vi "介面改良.vi"() -> ()   [LabVIEW 2022 SP3]
uses:
  <vilib>/httpClient/LabVIEWHTTPClient.lvlib
panel:
  in  "stop":bool
  in  "開始運作":bool
  out "異常指示燈":bool
  out "目前溫度":dbl
  in  "-10":bool
  in  "-5":bool
  in  "+5":bool
  in  "+10":bool
  out "目標溫度控制":string
  in  "溫差容許值":dbl
  in  "目標溫度":dbl
  in  "進階選單":bool
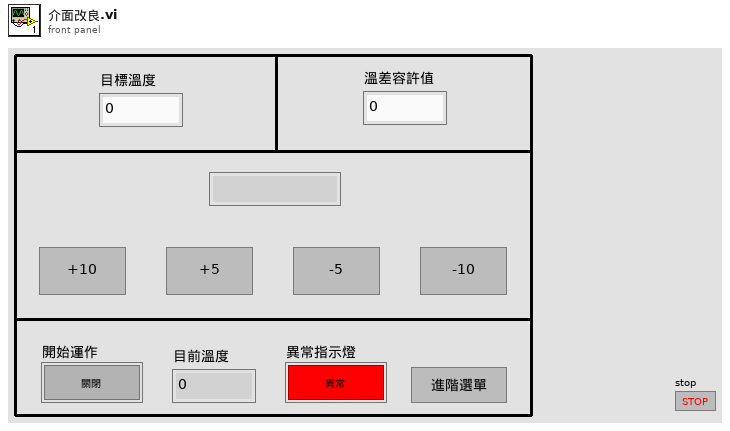
[diagram p1: front panel]
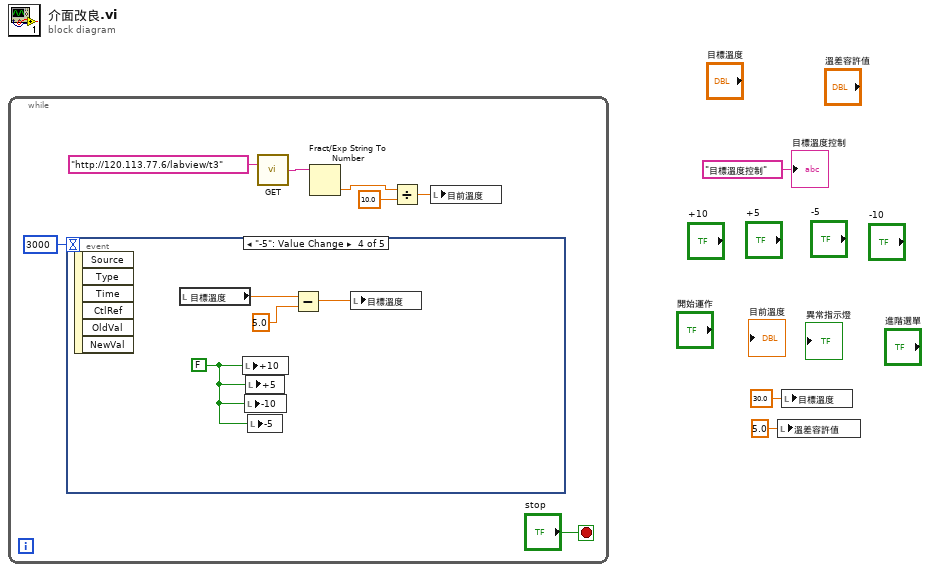
[diagram p0: block diagram]
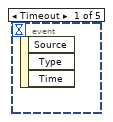
[diagram p2: hidden frame]
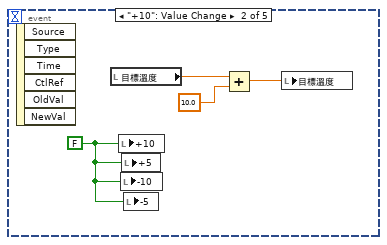
[diagram p3: hidden frame]
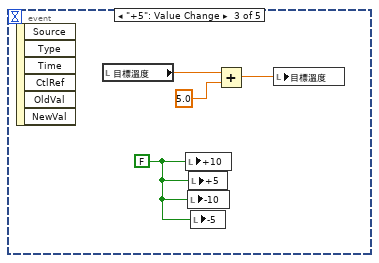
[diagram p4: hidden frame]
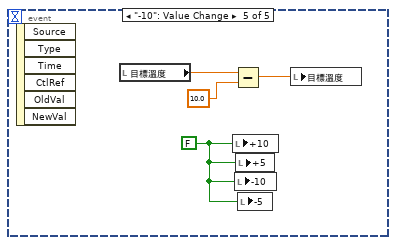
[diagram p5: hidden frame]
diagram:
  n1 = while {
    stop <- "stop" stop-if-true
    n2 = event shown="[3] \"-5\": Value Change" {
      selector: _ -> [_ _ _ _ _]
      dyn-events: _ -> [_ _ _ _ _]
      timeout: 3000 -> [_ _ _ _ _]
      event Timeout {
        n3 = event-data() -> ()  [unwired: 1 in, 3 out]
      }
      event "+10": Value Change {
        w11 = FALSE ("+10")
        n4 = event-data() -> ()  [unwired: 1 in, 6 out]
        n5 = local read "目標溫度"() -> (w12:dbl)
        n6 = local write "+10"(w11) -> ()
        n7 = local write "-10"(w11) -> ()
        n8 = local write "+5"(w11) -> ()
        n9 = local write "-5"(w11) -> ()
        n10 = Add(x=w12, y=10.0) -> (x+y=w14:dbl)
        n11 = local write "目標溫度"(w14) -> ()
      }
      event "+5": Value Change {
        w18 = FALSE ("+10")
        n12 = event-data() -> ()  [unwired: 1 in, 6 out]
        n13 = local read "目標溫度"() -> (w15:dbl)
        n14 = local write "+10"(w18) -> ()
        n15 = local write "-10"(w18) -> ()
        n16 = local write "+5"(w18) -> ()
        n17 = local write "-5"(w18) -> ()
        n18 = Add(x=w15, y=5.0) -> (x+y=w17:dbl)
        n19 = local write "目標溫度"(w17) -> ()
      }
      event "-5": Value Change {
        w19 = FALSE ("+10")
        n20 = event-data() -> ()  [unwired: 1 in, 6 out]
        n21 = local read "目標溫度"() -> (w20:dbl)
        n22 = local write "+10"(w19) -> ()
        n23 = local write "-10"(w19) -> ()
        n24 = local write "+5"(w19) -> ()
        n25 = local write "-5"(w19) -> ()
        n26 = Subtract(x=w20, y=5.0) -> (x-y=w21:dbl)
        n27 = local write "目標溫度"(w21) -> ()
      }
      event "-10": Value Change {
        w23 = FALSE ("+10")
        n28 = event-data() -> ()  [unwired: 1 in, 6 out]
        n29 = local read "目標溫度"() -> (w24:dbl)
        n30 = Subtract(x=w24, y=10.0) -> (x-y=w25:dbl)
        n31 = local write "+10"(w23) -> ()
        n32 = local write "-10"(w23) -> ()
        n33 = local write "+5"(w23) -> ()
        n34 = local write "-5"(w23) -> ()
        n35 = local write "目標溫度"(w25) -> ()
      }
    }
    n36 = call <vilib>:"GET.vi"("url"="http://120.113.77.6/labview/t3") -> ("body"=w10:string)  [unwired: 11 in, 3 out]
    n37 = Fract/Exp String To Number(string=w10) -> (number=w8:dbl)  [unwired: 3 in, 1 out]
    n38 = Divide(x=w8, y=10.0) -> (x/y=w5:dbl)
    n39 = local write "目前溫度"(w5) -> ()
  }
  n40 = local write "溫差容許值"(5.0 ("溫差容許值")) -> ()
  n41 = local write "目標溫度"(30.0 ("目標溫度")) -> ()
  "目標溫度控制" <- "目標溫度控制" ("目標溫度控制")
